vi "Stop Core.vi"(10 "final error code":i32, 11 "SM140 Actor in":refnum<class "SM140 Actor.lvclass">) -> (3 "SM140 Actor out":refnum<class "SM140 Actor.lvclass">)   [LabVIEW 2017, in "SM140.lvlib" / "SM140 Actor.lvclass"]
doc: "In addition to the following, this method also sends a message to the monitor to notify it that the actor has stopped execution.\n\n(<B>Filename</B>: Actor Framework.lvlib:Actor.lvclass:Stop Core.vi)\n\nDefines what the actor does before it stops. Use the <B>final error code</B> input to determine whether the actor shut down in response to an error.\n\nBy default, this method does nothing. A descendant class may override it to define behavior, such as shutting down any processes the actor initiated in its override of the Actor Core method.\n\nCopyright: MGI\nAuthored by: Derek Trepanier"
uses:
  SM140 Actor.lvclass
  SM140 Actor.lvclass/SM140 Actor.ctl
  Actor Monitor/Actor/Monitored Actor.lvclass
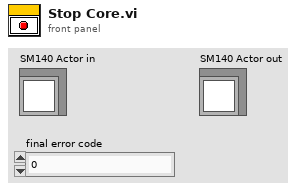
[diagram p1: front panel]
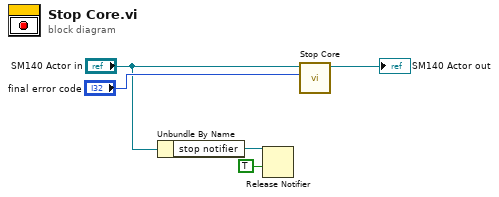
[diagram p0: block diagram]
diagram:
  n1 = Unbundle By Name("SM140 Actor in") -> ("stop notifier"=w2:refnum<notifier>)
  n2 = Release Notifier(notifier=w2, force destroy? (F)=TRUE) -> ()  [unwired: 1 in, 3 out]
  n3 = call-parent "Stop Core.vi"("final error code"="final error code", "Monitored Actor in"="SM140 Actor in") -> ("Monitored Actor out"=→"SM140 Actor out":refnum<class "SM140 Actor.lvclass">)  [unwired: 9 in]
